vi "Begin.vi"(8 "error in":errorcluster) -> (0 "error out":errorcluster)   [LabVIEW 2019]
doc: "Called before other user functions, this VI can be used to open I/O refnums, load in file data, and do general program initialization. Notice that the <B>error out</B> terminal is simply used for data flow. Wiring it to other structures or subVIs ensures that this VI runs first."
uses:
  <vilib>/Rock Robotics/WPI/DriverStation/WPI_DriverStationRobotMode2.ctl
  <vilib>/Rock Robotics/WPI/Joystick/WPI_JoystickDeviceEnum.ctl
  <vilib>/Rock Robotics/SystemInterfaces/DIO/FPGA_DIOPWMChannel.ctl
  <vilib>/Rock Robotics/WPI/SafetyOutput/WPI_SafetyOutputConfigMenu.ctl
  <vilib>/Rock Robotics/WPI/Solenoid/WPI_SolenoidChannel.ctl
  <vilib>/Rock Robotics/WPI/Solenoid/WPI_SolenoidValue.ctl
  <vilib>/Rock Robotics/SystemInterfaces/i2clib/i2c_bus.ctl
  Robot Global Data.vi
  <vilib>/Rock Robotics/WPI/MotorControl/WPI_MotorControlOpen SPARK.vi
  <vilib>/Rock Robotics/WPI/Solenoid/WPI_SolenoidOpenDouble.vi
  <vilib>/Rock Robotics/WPI/Solenoid/WPI_SolenoidSetEnum.vi
  <vilib>/Rock Robotics/Network Tables/NT Write Number.vi
  <vilib>/Rock Robotics/WPI/RobotDrive/WPI_RobotDriveOpen2MotorWithExistingMotors.vi
  <vilib>/Rock Robotics/Network Tables/NT Write Numeric Array.vi
  <vilib>/Rock Robotics/Network Tables/NT Write Boolean Array.vi
panel:
  in  "Blue Calibration":cluster{"R":dbl, "G":dbl, "B":dbl}={"R"=0.143, "G"=0.427, "B"=0.429}
  in  "Green Calibration":cluster{"R":dbl, "G":dbl, "B":dbl}={"R"=0.197, "G"=0.561, "B"=0.24}
  in  "Red Calibration":cluster{"R":dbl, "G":dbl, "B":dbl}={"R"=0.561, "G"=0.323, "B"=0.114}
  in  "Yellow Calibration":cluster{"R":dbl, "G":dbl, "B":dbl}={"R"=0.361, "G"=0.524, "B"=0.113}
  in  "Calibration Time (sec)":u32=4
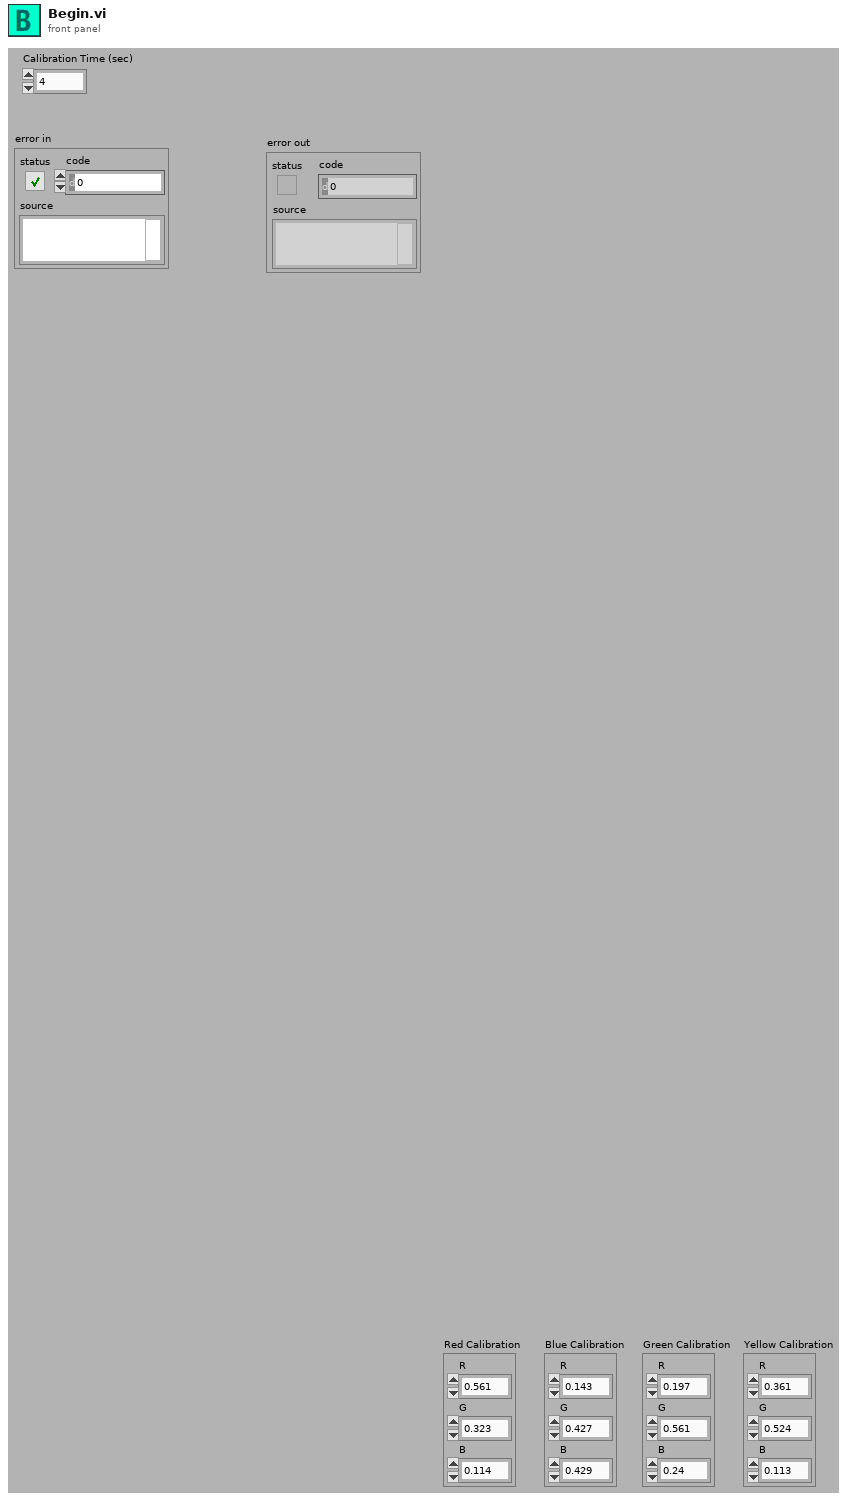
[diagram p1: front panel]
types:
  T1 = typedef "WPI_SolenoidChannel.ctl" = enum8{"Solenoid 0", "Solenoid 1", "Solenoid 2", "Solenoid 3", "Solenoid 4", "Solenoid 5", "Solenoid 6", "Solenoid 7", "Invalid"}
  T2 = typedef "WPI_SolenoidValue.ctl" = enum16{"Off", "On", "Forward", "Reverse"}
  T3 = typedef "WPI_SafetyOutputConfigMenu.ctl" = enum16{"Enable", "Disable"}
  T4 = typedef "i2c_bus.ctl" = enum16{"I2C On-Board", "I2C MXP", "Invalid"}
  T5 = typedef "FPGA_DIOPWMChannel.ctl" = enum8{"PWM 0", "PWM 1", "PWM 2", "PWM 3", "PWM 4", "PWM 5", "PWM 6", "PWM 7", "PWM 8", "PWM 9", "PWM MXP 0", "PWM MXP 1", "PWM MXP 2", "PWM MXP 3", "PWM MXP 4", "PWM MXP 5", "PWM MXP 6", "PWM MXP 7", "PWM MXP 8", "PWM MXP 9", "Invalid"}
  T6 = typedef "WPI_JoystickDeviceEnum.ctl" = enum16{"USB 0", "USB 1", "USB 2", "USB 3", "USB 4", "USB 5"}
  T7 = typedef "WPI_DriverStationRobotMode2.ctl" = enum16{"Autonomous Disabled", "Autonomous Enabled", "Teleop Disabled", "Teleop Enabled", "Disconnected", "Finish", "Test Disabled", "Test Enabled", "Emergency Stopped"}
  T8 = typedef "WPI_JoystickDevRef.ctl" = cluster{"Device":T6}
  T9 = typedef "WPI_MotorControlDeviceRef.ctl" = cluster{"DeviceStatus":errorcluster, "Type":T10, "PWM":cluster{"PWM Channel":T5, "DeadBand":T11}, "CAN":cluster{"Device Number":u8, "SetOutput VI Ref":variant, "GetOutput VI Ref":variant, "Enable VI Ref":variant, "Disable VI Ref":variant, "Data":variant}, "Invert":bool, "DIO PWM":cluster{"PWM \"Enable\" Channel":T5, "DIOChannel":T12, "PWM Rate":dbl}}
  T10 = typedef "WPI_MotorControlType.ctl" = enum16{"PWM", "CAN", "DIO PWM"}
  T11 = typedef "WPI_PWMDeadband.ctl" = cluster{"Name":string, "maxPositivePwm":i32, "minPositivePwm":i32, "centerPwm":i32, "maxNegativePwm":i32, "minNegativePwm":i32, "angularRange":u16}
  T12 = typedef "FPGA_DIOChannel.ctl" = enum8{"DIO 0", "DIO 1", "DIO 2", "DIO 3", "DIO 4", "DIO 5", "DIO 6", "DIO 7", "DIO 8", "DIO 9", "DIO MXP 0", "DIO MXP 1", "DIO MXP 2", "DIO MXP 3", "DIO MXP 4", "DIO MXP 5", "DIO MXP 6", "DIO MXP 7", "DIO MXP 8", "DIO MXP 9", "DIO MXP 10", "DIO MXP 11", "DIO MXP 12", "DIO MXP 13", "DIO MXP 14", "DIO MXP 15", "SPI Port CS1", "SPI Port CS2", "SPI Port CS3", "SPI Port MISO", "SPI Port MOSI", "Invalid"}
  T13 = typedef "WPI_RobotDriveDevRef.ctl" = cluster{"DevStatus":errorcluster, "Motors[]":T9[], "Square Inputs":bool, "Max Output":dbl}
  T14 = typedef "ADIS 16448 HW Configuration.ctl" = cluster{"SPI Clock Rate (Hz)":dbl, "IMU SPI Mode (3)":T15, "IMU Reset Pin":T12, "IMU SPI Bus":T16, "IMU Data Ready Pin":T12, "Stall Config":cluster{"Pow2BytesPerRead":u8, "StallTicks":u16, "CsToSclkTicks":u8}, "IMU Status LED Pin":T12}
  T15 = typedef "WPI_SPIMode.ctl" = enum16{"Mode 0 (Clk Idle Low,Sample on Leading)", "Mode 1 (Clk Idle Low,Sample on Trailing)", "Mode 2 (Clk Idle High,Sample on Leading)", "Mode 3 (Clk Idle High,Sample on Trailing)"}
  T16 = typedef "spi_bus.ctl" = enum16{"SPI On-Board, CS0", "SPI On-Board, CS1", "SPI On-Board, CS2", "SPI On-Board, CS3", "SPI MXP", "Invalid"}
  T17 = typedef "Color Sensor V3 DevRef.ctl" = cluster{"I2CDevRef":T18}
  T18 = typedef "WPI_I2CDevRef.ctl" = cluster{"DevStatus":errorcluster, "Device Address":u8, "Handle":i32, "I2C Bus":T4}
  T19 = typedef "WPI_SolenoidDevRef.ctl" = cluster{"DevStatus":errorcluster, "Pneumatics Control Module":u8, "Forward Solenoid Channel":T1, "Reverse Solenoid Channel":T1}
  T20 = typedef "ADIS16448 Device Reference.ctl" = cluster{"DevStatus":errorcluster, "Hardware Config":T21, "Calibration Complete":refnum<notifier>, "Status FIFO":refnum<k33>, "Last Value Reference":refnum<data-value>, "Sychronous Process VI":T22, "Cmd FIFO":refnum<k33>, "Source":T23, "Data FIFO":refnum<k33>, "IMU Status LED Pin":T12, "Calibration Time":u32}
  T21 = typedef "ADIS16448 Hardware Configuration.ctl" = cluster{"SPI Clock Rate (Hz)":dbl, "IMU SPI Mode (3)":T15, "IMU Reset Pin":T12, "IMU SPI Bus":T16, "IMU Data Ready Pin":T12, "Stall Config":cluster{"Pow2BytesPerRead":u8, "StallTicks":u16, "CsToSclkTicks":u8}, "IMU Status LED Pin":T12}
  T22 = typedef "ADIS16448 Process.ctl" = refnum<vi>
  T23 = typedef "FPGA_CounterEncoderSourceConvertionLVSourceType.ctl" = cluster{"DevStatus":errorcluster, "AnalogTriggerMode?":bool, "DigitalMode":cluster{"DIO Channel":T24}, "AnalogTriggerMode":cluster{"AnalogTriggerIndex":T25, "OutputType":T26}}
  T24 = typedef "FPGA_DIODigitalSourceChannel.ctl" = enum8{"DIO 0", "DIO 1", "DIO 2", "DIO 3", "DIO 4", "DIO 5", "DIO 6", "DIO 7", "DIO 8", "DIO 9", "DIO MXP 0", "DIO MXP 1", "DIO MXP 2", "DIO MXP 3", "DIO MXP 4", "DIO MXP 5", "DIO MXP 6", "DIO MXP 7", "DIO MXP 8", "DIO MXP 9", "DIO MXP 10", "DIO MXP 11", "DIO MXP 12", "DIO MXP 13", "DIO MXP 14", "DIO MXP 15", "SPI Port CS1", "SPI Port CS2", "SPI Port CS3", "SPI Port MISO", "SPI Port MOSI", "Disabled"}
  T25 = typedef "FPGA_AnalogTriggerIndex.ctl" = enum8{"Trig 0", "Trig 1", "Trig 2", "Trig 3", "Trig 4", "Trig 5", "Trig 6", "Trig 7", "Invalid"}
  T26 = typedef "FPGA_AnalogTriggerOutType.ctl" = enum16{"InWindow", "TriggerState", "Rising", "Falling"}
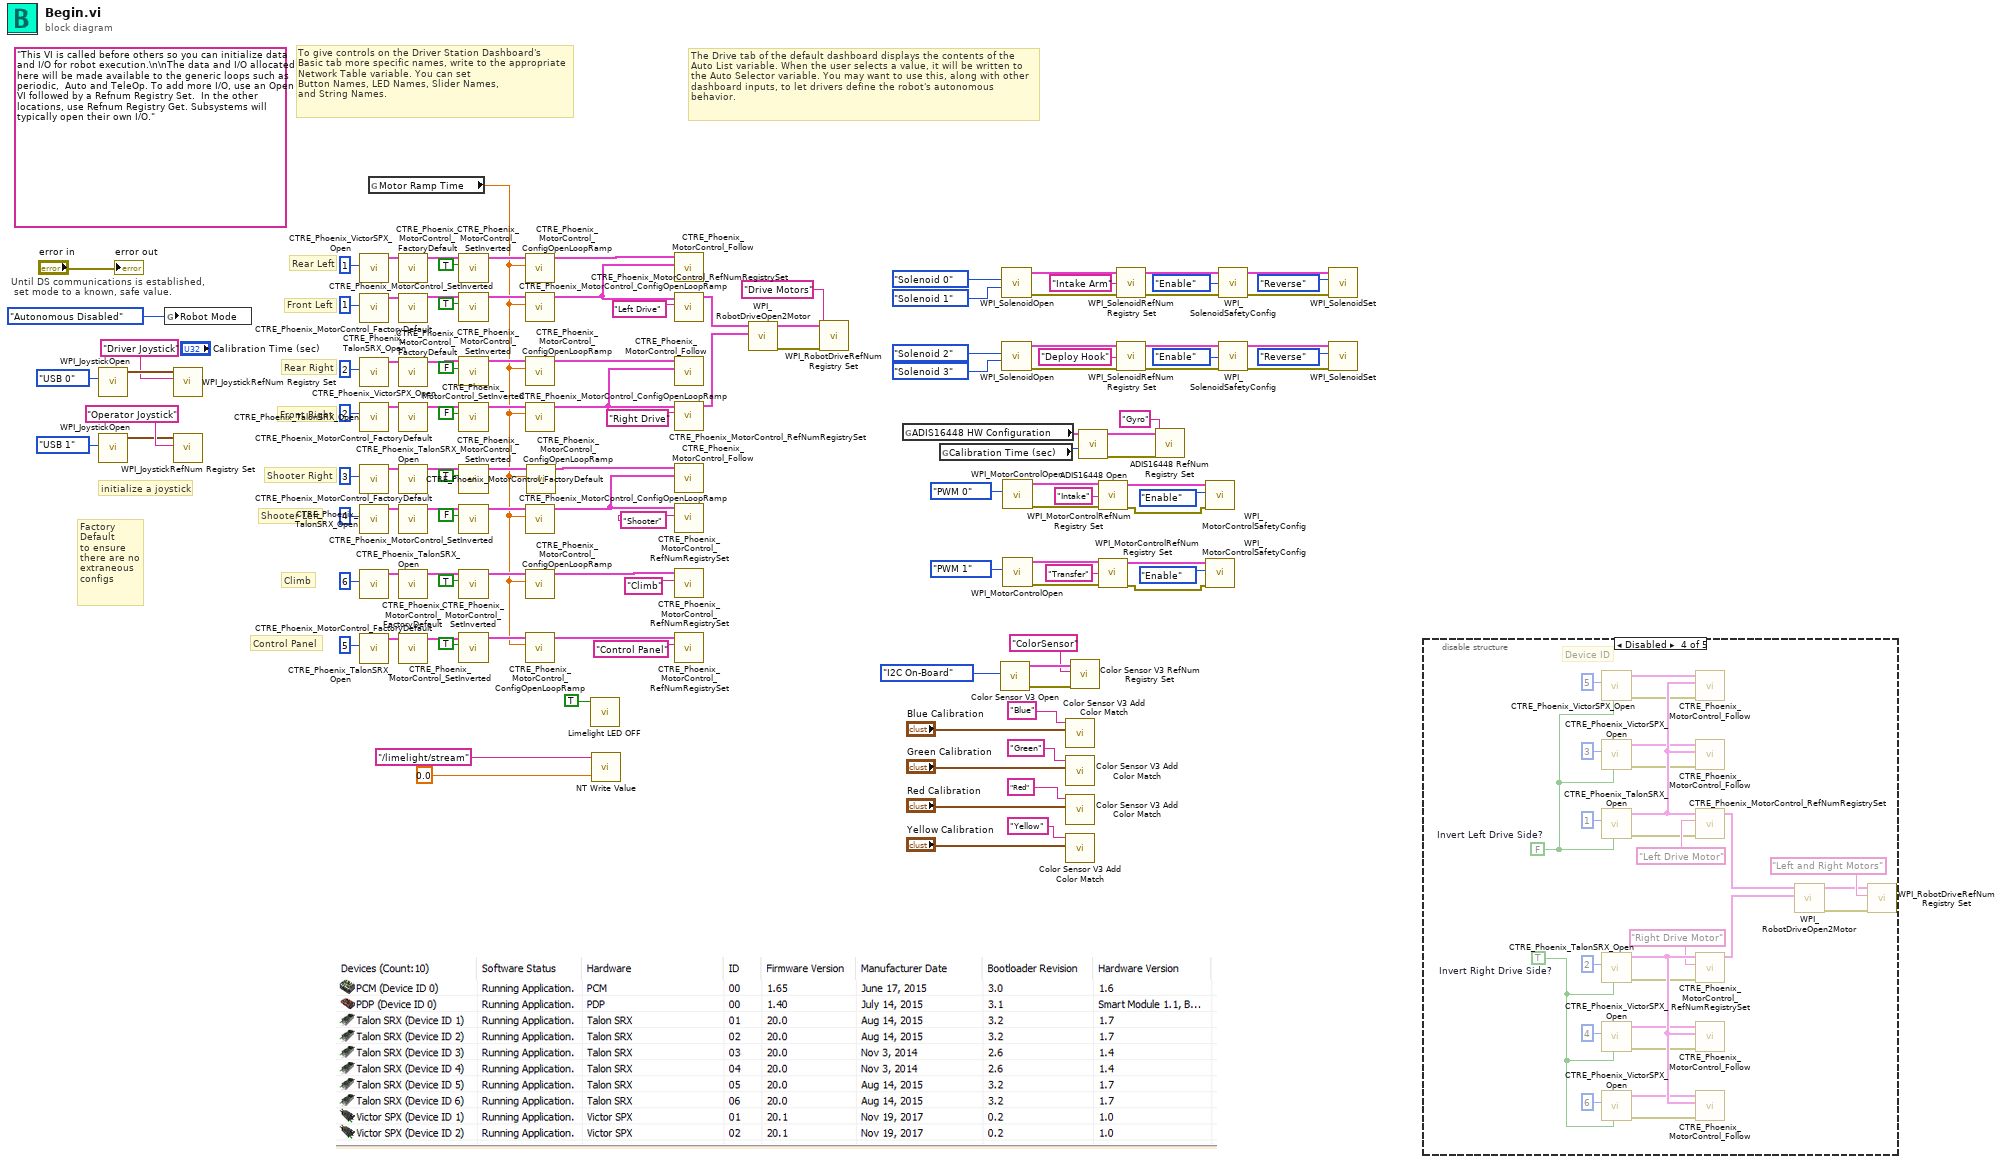
[diagram p0: block diagram]
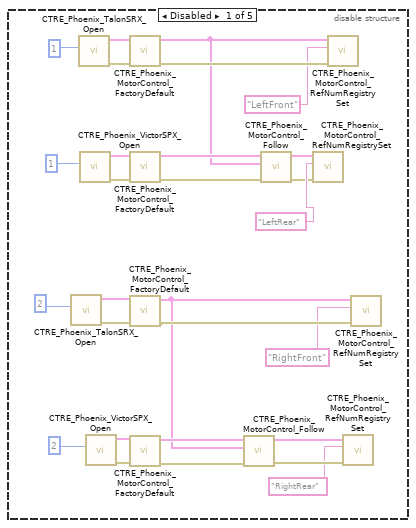
[diagram p2: hidden frame]
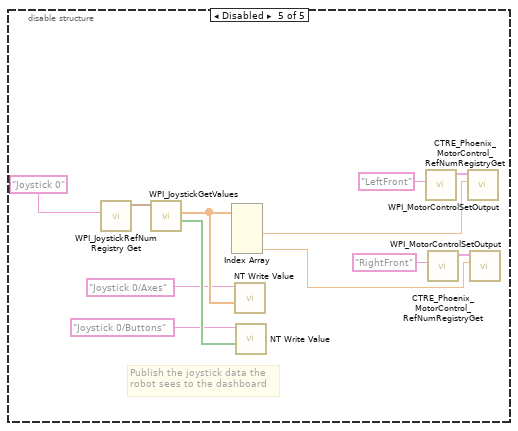
[diagram p5: hidden frame]
diagram:
  (unwired) "This VI is called before others so you can initialize data and I/O for robot execution.\n\nThe data and I/O allocated here will be made available to the generic loops such as periodic,  Auto and TeleOp. To add more I/O, use an Open VI followed by a Refnum Registry Set.  In the other locations, use Refnum Registry Get. Subsystems will typically open their own I/O."
  # "Climb"
  # "Control Panel"
  # "The Drive tab of the default dashboard displays the contents of the\nAuto List variable. When the user selects a value, it will be written to\nthe Auto Selector variable. You may want to use this, along with other\ndashboard inputs, to let drivers define the robot's autonomous\nbehavior."
  # "To give controls on the Driver Station Dashboard's\nBasic tab more specific names, write to the appropriate\nNetwork Table variable. You can set\nButton Names, LED Names, Slider Names,\nand String Names."
  # "Shooter Left"
  # "Shooter Right"
  # "Factory \nDefault \nto ensure \nthere are no \nextraneous \nconfigs"
  # "Front Right"
  # "Front Left"
  # "Rear Right"
  # "Rear Left"
  # "initialize a joystick"
  # "Until DS communications is established,\n set mode to a known, safe value."
  n1 = call <vilib>:"WPI_JoystickOpen.vi"("JoystickDevice"=WPI_JoystickDeviceEnum."USB 0") -> ("JoystickDevRef"=w106:T8)  [unwired: 10 in]
  n2 = call <vilib>:"WPI_JoystickOpen.vi"("JoystickDevice"=WPI_JoystickDeviceEnum."USB 1") -> ("JoystickDevRef"=w121:T8)  [unwired: 10 in]
  n3 = global write "Robot Global Data.vi" "Robot Mode"(WPI_DriverStationRobotMode2."Autonomous Disabled" ("Robot Mode")) -> ()
  n4 = call <vilib>:"WPI_JoystickRefNum Registry Set.vi"("refnum name"="Driver Joystick", "JoystickDevRef"=w106) -> ()  [unwired: 8 in, 2 out]
  n5 = call <vilib>:"WPI_JoystickRefNum Registry Set.vi"("refnum name"="Operator Joystick", "JoystickDevRef"=w121) -> ()  [unwired: 8 in, 2 out]
  n6 = call <vilib>:"CTRE_Phoenix_VictorSPX_Open.vi"("Device Number"=u8 1) -> ("CAN Talon SRX Ref"=w104:T9)  [unwired: 9 in, 1 out]
  n7 = call <vilib>:"CTRE_Phoenix_TalonSRX_Open.vi"("Device Number"=u8 1) -> ("CAN Talon SRX Ref"=w103:T9)  [unwired: 9 in, 1 out]
  n8 = call <vilib>:"CTRE_Phoenix_VictorSPX_Open.vi"("Device Number"=u8 2) -> ("CAN Talon SRX Ref"=w102:T9)  [unwired: 9 in, 1 out]
  n9 = call <vilib>:"CTRE_Phoenix_TalonSRX_Open.vi"("Device Number"=u8 2) -> ("CAN Talon SRX Ref"=w101:T9)  [unwired: 9 in, 1 out]
  n10 = call <vilib>:"CTRE_Phoenix_TalonSRX_Open.vi"("Device Number"=u8 3) -> ("CAN Talon SRX Ref"=w75:T9)  [unwired: 9 in, 1 out]
  n11 = call <vilib>:"CTRE_Phoenix_TalonSRX_Open.vi"("Device Number"=u8 4) -> ("CAN Talon SRX Ref"=w74:T9)  [unwired: 9 in, 1 out]
  n12 = call <vilib>:"CTRE_Phoenix_TalonSRX_Open.vi"("Device Number"=u8 6) -> ("CAN Talon SRX Ref"=w26:T9)  [unwired: 9 in, 1 out]
  n13 = call <vilib>:"CTRE_Phoenix_TalonSRX_Open.vi"("Device Number"=u8 5) -> ("CAN Talon SRX Ref"=w56:T9)  [unwired: 9 in, 1 out]
  n14 = global read "Robot Global Data.vi" "Motor Ramp Time"() -> (w1:dbl)
  n15 = call <vilib>:"CTRE_Phoenix_MotorControl_FactoryDefault.vi"("PhoenixMotorControlDevRef"=w104) -> ("PhoenixMotorControlDevRef"=w99:T9)  [unwired: 9 in, 1 out]
  n16 = call <vilib>:"CTRE_Phoenix_MotorControl_FactoryDefault.vi"("PhoenixMotorControlDevRef"=w103) -> ("PhoenixMotorControlDevRef"=w97:T9)  [unwired: 9 in, 1 out]
  n17 = call <vilib>:"CTRE_Phoenix_MotorControl_FactoryDefault.vi"("PhoenixMotorControlDevRef"=w102) -> ("PhoenixMotorControlDevRef"=w95:T9)  [unwired: 9 in, 1 out]
  n18 = call <vilib>:"CTRE_Phoenix_MotorControl_FactoryDefault.vi"("PhoenixMotorControlDevRef"=w101) -> ("PhoenixMotorControlDevRef"=w93:T9)  [unwired: 9 in, 1 out]
  n19 = call <vilib>:"CTRE_Phoenix_MotorControl_FactoryDefault.vi"("PhoenixMotorControlDevRef"=w75) -> ("PhoenixMotorControlDevRef"=w72:T9)  [unwired: 9 in, 1 out]
  n20 = call <vilib>:"CTRE_Phoenix_MotorControl_FactoryDefault.vi"("PhoenixMotorControlDevRef"=w74) -> ("PhoenixMotorControlDevRef"=w70:T9)  [unwired: 9 in, 1 out]
  n21 = call <vilib>:"CTRE_Phoenix_MotorControl_FactoryDefault.vi"("PhoenixMotorControlDevRef"=w26) -> ("PhoenixMotorControlDevRef"=w24:T9)  [unwired: 9 in, 1 out]
  n22 = call <vilib>:"CTRE_Phoenix_MotorControl_FactoryDefault.vi"("PhoenixMotorControlDevRef"=w56) -> ("PhoenixMotorControlDevRef"=w54:T9)  [unwired: 9 in, 1 out]
  n23 = call <vilib>:"CTRE_Phoenix_MotorControl_SetInverted.vi"("Invert?"=TRUE, "PhoenixMotorControlDevRef"=w99) -> ("PhoenixMotorControlDevRef"=w17:T9)  [unwired: 8 in, 1 out]
  n24 = call <vilib>:"CTRE_Phoenix_MotorControl_SetInverted.vi"("Invert?"=TRUE, "PhoenixMotorControlDevRef"=w97) -> ("PhoenixMotorControlDevRef"=w15:T9)  [unwired: 8 in, 1 out]
  n25 = call <vilib>:"CTRE_Phoenix_MotorControl_SetInverted.vi"("Invert?"=FALSE, "PhoenixMotorControlDevRef"=w95) -> ("PhoenixMotorControlDevRef"=w9:T9)  [unwired: 8 in, 1 out]
  n26 = call <vilib>:"CTRE_Phoenix_MotorControl_SetInverted.vi"("Invert?"=FALSE, "PhoenixMotorControlDevRef"=w93) -> ("PhoenixMotorControlDevRef"=w10:T9)  [unwired: 8 in, 1 out]
  n27 = call <vilib>:"CTRE_Phoenix_MotorControl_SetInverted.vi"("Invert?"=TRUE, "PhoenixMotorControlDevRef"=w72) -> ("PhoenixMotorControlDevRef"=w3:T9)  [unwired: 8 in, 1 out]
  n28 = call <vilib>:"CTRE_Phoenix_MotorControl_SetInverted.vi"("Invert?"=FALSE, "PhoenixMotorControlDevRef"=w70) -> ("PhoenixMotorControlDevRef"=w11:T9)  [unwired: 8 in, 1 out]
  n29 = call <vilib>:"CTRE_Phoenix_MotorControl_SetInverted.vi"("Invert?"=TRUE, "PhoenixMotorControlDevRef"=w24) -> ("PhoenixMotorControlDevRef"=w12:T9)  [unwired: 8 in, 1 out]
  n30 = call <vilib>:"CTRE_Phoenix_MotorControl_SetInverted.vi"("Invert?"=TRUE, "PhoenixMotorControlDevRef"=w54) -> ("PhoenixMotorControlDevRef"=w13:T9)  [unwired: 8 in, 1 out]
  n31 = call <vilib>:"CTRE_Phoenix_MotorControl_ConfigOpenLoopRamp.vi"("secondsFromNeutralToFull"=w1, "PhoenixMotorControlDevRef"=w17) -> ("PhoenixMotorControlDevRef"=w16:T9)  [unwired: 8 in, 1 out]
  n32 = call <vilib>:"CTRE_Phoenix_MotorControl_ConfigOpenLoopRamp.vi"("secondsFromNeutralToFull"=w1, "PhoenixMotorControlDevRef"=w15) -> ("PhoenixMotorControlDevRef"=w14:T9)  [unwired: 8 in, 1 out]
  n33 = call <vilib>:"CTRE_Phoenix_MotorControl_ConfigOpenLoopRamp.vi"("secondsFromNeutralToFull"=w1, "PhoenixMotorControlDevRef"=w9) -> ("PhoenixMotorControlDevRef"=w8:T9)  [unwired: 8 in, 1 out]
  n34 = call <vilib>:"CTRE_Phoenix_MotorControl_ConfigOpenLoopRamp.vi"("secondsFromNeutralToFull"=w1, "PhoenixMotorControlDevRef"=w10) -> ("PhoenixMotorControlDevRef"=w7:T9)  [unwired: 8 in, 1 out]
  n35 = call <vilib>:"CTRE_Phoenix_MotorControl_ConfigOpenLoopRamp.vi"("secondsFromNeutralToFull"=w1, "PhoenixMotorControlDevRef"=w11) -> ("PhoenixMotorControlDevRef"=w6:T9)  [unwired: 8 in, 1 out]
  n36 = call <vilib>:"CTRE_Phoenix_MotorControl_ConfigOpenLoopRamp.vi"("secondsFromNeutralToFull"=w1, "PhoenixMotorControlDevRef"=w12) -> ("PhoenixMotorControlDevRef"=w5:T9)  [unwired: 8 in, 1 out]
  n37 = call <vilib>:"CTRE_Phoenix_MotorControl_ConfigOpenLoopRamp.vi"("secondsFromNeutralToFull"=w1, "PhoenixMotorControlDevRef"=w13) -> ("PhoenixMotorControlDevRef"=w4:T9)  [unwired: 8 in, 1 out]
  n38 = call <vilib>:"CTRE_Phoenix_MotorControl_ConfigOpenLoopRamp.vi"("secondsFromNeutralToFull"=w1, "PhoenixMotorControlDevRef"=w3) -> ("PhoenixMotorControlDevRef"=w2:T9)  [unwired: 8 in, 1 out]
  n39 = call "Limelight LED OFF.vi"("D Select  8"=TRUE) -> ()  [unwired: 10 in, 1 out]
  n40 = call-poly <vilib>:"NT Write Value.vi"("Numeric"=0.0, "Name"="/limelight/stream") -> ()  [unwired: 9 in, 1 out]
  n41 = call <vilib>:"CTRE_Phoenix_MotorControl_Follow.vi"("Master Controller to Follow"=w14, "PhoenixMotorControlDevRef"=w16) -> ()  [unwired: 8 in, 2 out]
  n42 = call <vilib>:"CTRE_Phoenix_MotorControl_RefNumRegistrySet.vi"("refnum name"="Left Drive", "PhoenixMotorControlDevRef"=w14) -> ("PhoenixMotorControlDevRef"=w114:T9)  [unwired: 8 in, 1 out]
  n43 = call <vilib>:"CTRE_Phoenix_MotorControl_Follow.vi"("Master Controller to Follow"=w7, "PhoenixMotorControlDevRef"=w8) -> ()  [unwired: 8 in, 2 out]
  n44 = call <vilib>:"CTRE_Phoenix_MotorControl_RefNumRegistrySet.vi"("refnum name"="Right Drive", "PhoenixMotorControlDevRef"=w7) -> ("PhoenixMotorControlDevRef"=w113:T9)  [unwired: 8 in, 1 out]
  n45 = call <vilib>:"CTRE_Phoenix_MotorControl_Follow.vi"("Master Controller to Follow"=w6, "PhoenixMotorControlDevRef"=w2) -> ()  [unwired: 8 in, 2 out]
  n46 = call <vilib>:"CTRE_Phoenix_MotorControl_RefNumRegistrySet.vi"("refnum name"="Shooter", "PhoenixMotorControlDevRef"=w6) -> ()  [unwired: 8 in, 2 out]
  n47 = call <vilib>:"CTRE_Phoenix_MotorControl_RefNumRegistrySet.vi"("refnum name"="Climb", "PhoenixMotorControlDevRef"=w5) -> ()  [unwired: 8 in, 2 out]
  n48 = call <vilib>:"CTRE_Phoenix_MotorControl_RefNumRegistrySet.vi"("refnum name"="Control Panel", "PhoenixMotorControlDevRef"=w4) -> ()  [unwired: 8 in, 2 out]
  n49 = call-poly <vilib>:"WPI_RobotDriveOpen2Motor.vi"("Right Motor Dev Ref"=w113, "Left Motor Dev Ref"=w114) -> ("error out"=w109:errorcluster, "RobotDriveDevRef"=w110:T13)  [unwired: 8 in]
  n50 = call <vilib>:"WPI_RobotDriveRefNum Registry Set.vi"("error in (no error)"=w109, "refnum name"="Drive Motors", "RobotDriveDevRef"=w110) -> ()  [unwired: 7 in, 2 out]
  n51 = global read "Robot Global Data.vi" "ADIS16448 HW Configuration"() -> (w22:T14)
  n52 = global read "Robot Global Data.vi" "Calibration Time (sec)"() -> (w21:u32)
  n53 = call <vilib>:"Color Sensor V3 Open.vi"("I2C Bus"=i2c_bus."I2C On-Board") -> ("error out"=w51:errorcluster, "ColorSensorDevRef"=w52:T17)  [unwired: 9 in]
  n54 = call-poly <vilib>:"WPI_SolenoidOpen.vi"("Reverse Solenoid Channel"=WPI_SolenoidChannel."Solenoid 1" ("Solenoid Channel"), "Forward Solenoid Channel"=WPI_SolenoidChannel."Solenoid 0" ("Solenoid Channel")) -> ("error out"=w66:errorcluster, "SolenoidDevRef"=w69:T19)  [unwired: 8 in]
  n55 = call-poly <vilib>:"WPI_SolenoidOpen.vi"("Reverse Solenoid Channel"=WPI_SolenoidChannel."Solenoid 3" ("Solenoid Channel"), "Forward Solenoid Channel"=WPI_SolenoidChannel."Solenoid 2" ("Solenoid Channel")) -> ("error out"=w33:errorcluster, "SolenoidDevRef"=w30:T19)  [unwired: 8 in]
  n56 = call-poly <vilib>:"WPI_MotorControlOpen.vi"("PWM Channel"=FPGA_DIOPWMChannel."PWM 0") -> ("error out"=w87:errorcluster, "MotorControlDeviceRef"=w91:T9)  [unwired: 9 in]
  n57 = call-poly <vilib>:"WPI_MotorControlOpen.vi"("PWM Channel"=FPGA_DIOPWMChannel."PWM 1") -> ("error out"=w84:errorcluster, "MotorControlDeviceRef"=w80:T9)  [unwired: 9 in]
  n58 = call <vilib>:"Color Sensor V3 Add Color Match.vi"("Color"="Blue Calibration", "Name"="Blue") -> ()  [unwired: 10 in]
  n59 = call <vilib>:"Color Sensor V3 Add Color Match.vi"("Color"="Green Calibration", "Name"="Green") -> ()  [unwired: 10 in]
  n60 = call <vilib>:"Color Sensor V3 Add Color Match.vi"("Color"="Red Calibration", "Name"="Red") -> ()  [unwired: 10 in]
  n61 = call <vilib>:"Color Sensor V3 Add Color Match.vi"("Color"="Yellow Calibration", "Name"="Yellow") -> ()  [unwired: 10 in]
  n62 = call <vilib>:"Color Sensor V3 RefNum Registry Set.vi"("error in (no error)"=w51, "refnum name"="ColorSensor", "ColorSensorDevRef"=w52) -> ()  [unwired: 7 in, 2 out]
  n63 = call <vilib>:"ADIS16448 Open.vi"("Initial Calibration Time (sec)"=w21, "Hardware Config"=w22) -> ("error out"=w19:errorcluster, "ADIS16448DevRef"=w20:T20)  [unwired: 8 in]
  n64 = call <vilib>:"WPI_MotorControlRefNum Registry Set.vi"("error in (no error)"=w87, "refnum name"="Intake", "MotorControlDevRef"=w91) -> ("error out"=w86:errorcluster, "MotorControlDevRef"=w90:T9)  [unwired: 7 in]
  n65 = call <vilib>:"WPI_MotorControlRefNum Registry Set.vi"("error in (no error)"=w84, "refnum name"="Transfer", "MotorControlDevRef"=w80) -> ("error out"=w85:errorcluster, "MotorControlDevRef"=w81:T9)  [unwired: 7 in]
  n66 = call <vilib>:"WPI_SolenoidRefNum Registry Set.vi"("error in (no error)"=w66, "refnum name"="Intake Arm", "SolenoidDevRef"=w69) -> ("error out"=w65:errorcluster, "SolenoidDevRef"=w68:T19)  [unwired: 7 in]
  n67 = call <vilib>:"WPI_SolenoidRefNum Registry Set.vi"("error in (no error)"=w33, "refnum name"="Deploy Hook", "SolenoidDevRef"=w30) -> ("error out"=w34:errorcluster, "SolenoidDevRef"=w31:T19)  [unwired: 7 in]
  n68 = call <vilib>:"ADIS16448 RefNum Registry Set.vi"("error in (no error)"=w19, "refnum name"="Gyro", "ADIS16448DevRef"=w20) -> ()  [unwired: 7 in, 2 out]
  n69 = call <vilib>:"WPI_MotorControlSafetyConfig.vi"("error in (no error)"=w86, "mode"=WPI_SafetyOutputConfigMenu."Enable", "MotorControlDevRef"=w90) -> ()  [unwired: 7 in, 2 out]
  n70 = call <vilib>:"WPI_MotorControlSafetyConfig.vi"("error in (no error)"=w85, "mode"=WPI_SafetyOutputConfigMenu."Enable", "MotorControlDevRef"=w81) -> ()  [unwired: 7 in, 2 out]
  n71 = call <vilib>:"WPI_SolenoidSafetyConfig.vi"("error in (no error)"=w65, "mode"=WPI_SafetyOutputConfigMenu."Enable", "SolenoidDevRef"=w68) -> ("error out"=w64:errorcluster, "SolenoidDevRef"=w67:T19)  [unwired: 7 in]
  n72 = call <vilib>:"WPI_SolenoidSafetyConfig.vi"("error in (no error)"=w34, "mode"=WPI_SafetyOutputConfigMenu."Enable", "SolenoidDevRef"=w31) -> ("error out"=w35:errorcluster, "SolenoidDevRef"=w32:T19)  [unwired: 7 in]
  n73 = call-poly <vilib>:"WPI_SolenoidSet.vi"("error in (no error)"=w64, "Value"=WPI_SolenoidValue."Reverse", "SolenoidDevRef"=w67) -> ()  [unwired: 7 in, 2 out]
  n74 = call-poly <vilib>:"WPI_SolenoidSet.vi"("error in (no error)"=w35, "Value"=WPI_SolenoidValue."Reverse", "SolenoidDevRef"=w32) -> ()  [unwired: 7 in, 2 out]
  n75 = disable-structure shown="Disabled" {
    frame Disabled {
      n76 = call <vilib>:"CTRE_Phoenix_TalonSRX_Open.vi"("Device Number"=u8 2) -> ("error out"=w148:errorcluster, "CAN Talon SRX Ref"=w138:T9)  [unwired: 9 in]
      n77 = call <vilib>:"CTRE_Phoenix_TalonSRX_Open.vi"("Device Number"=u8 1) -> ("error out"=w146:errorcluster, "CAN Talon SRX Ref"=w136:T9)  [unwired: 9 in]
      n78 = call <vilib>:"CTRE_Phoenix_VictorSPX_Open.vi"("Device Number"=u8 1) -> ("error out"=w144:errorcluster, "CAN Talon SRX Ref"=w142:T9)  [unwired: 9 in]
      n79 = call <vilib>:"CTRE_Phoenix_VictorSPX_Open.vi"("Device Number"=u8 2) -> ("error out"=w150:errorcluster, "CAN Talon SRX Ref"=w140:T9)  [unwired: 9 in]
      n80 = call <vilib>:"CTRE_Phoenix_MotorControl_FactoryDefault.vi"("error in"=w146, "PhoenixMotorControlDevRef"=w136) -> ("error out"=w147:errorcluster, "PhoenixMotorControlDevRef"=w137:T9)  [unwired: 8 in]
      n81 = call <vilib>:"CTRE_Phoenix_MotorControl_FactoryDefault.vi"("error in"=w144, "PhoenixMotorControlDevRef"=w142) -> ("error out"=w145:errorcluster, "PhoenixMotorControlDevRef"=w143:T9)  [unwired: 8 in]
      n82 = call <vilib>:"CTRE_Phoenix_MotorControl_FactoryDefault.vi"("error in"=w148, "PhoenixMotorControlDevRef"=w138) -> ("error out"=w149:errorcluster, "PhoenixMotorControlDevRef"=w139:T9)  [unwired: 8 in]
      n83 = call <vilib>:"CTRE_Phoenix_MotorControl_FactoryDefault.vi"("error in"=w150, "PhoenixMotorControlDevRef"=w140) -> ("error out"=w151:errorcluster, "PhoenixMotorControlDevRef"=w141:T9)  [unwired: 8 in]
      n84 = call <vilib>:"CTRE_Phoenix_MotorControl_Follow.vi"("error in (no error)"=w151, "Master Controller to Follow"=w139, "PhoenixMotorControlDevRef"=w141) -> ("error out"=w134:errorcluster, "PhoenixMotorControlDevRef"=w135:T9)  [unwired: 7 in]
      n85 = call <vilib>:"CTRE_Phoenix_MotorControl_Follow.vi"("error in (no error)"=w145, "Master Controller to Follow"=w137, "PhoenixMotorControlDevRef"=w143) -> ("error out"=w126:errorcluster, "PhoenixMotorControlDevRef"=w127:T9)  [unwired: 7 in]
      n86 = call <vilib>:"CTRE_Phoenix_MotorControl_RefNumRegistrySet.vi"("error in (no error)"=w126, "refnum name"="LeftRear", "PhoenixMotorControlDevRef"=w127) -> ()  [unwired: 7 in, 2 out]
      n87 = call <vilib>:"CTRE_Phoenix_MotorControl_RefNumRegistrySet.vi"("error in (no error)"=w147, "refnum name"="LeftFront", "PhoenixMotorControlDevRef"=w137) -> ()  [unwired: 7 in, 2 out]
      n88 = call <vilib>:"CTRE_Phoenix_MotorControl_RefNumRegistrySet.vi"("error in (no error)"=w134, "refnum name"="RightRear", "PhoenixMotorControlDevRef"=w135) -> ()  [unwired: 7 in, 2 out]
      n89 = call <vilib>:"CTRE_Phoenix_MotorControl_RefNumRegistrySet.vi"("error in (no error)"=w149, "refnum name"="RightFront", "PhoenixMotorControlDevRef"=w139) -> ()  [unwired: 7 in, 2 out]
    }
    frame Enabled {
    }
    frame Disabled {
    }
    frame Disabled {
      w178 = FALSE  # Invert Left Drive Side?
      w177 = TRUE  # Invert Right Drive Side?
      # "Device ID"
      n90 = call <vilib>:"CTRE_Phoenix_VictorSPX_Open.vi"("Invert"=w178, "Device Number"=u8 5) -> ("error out"=w168:errorcluster, "CAN Talon SRX Ref"=w169:T9)  [unwired: 8 in]
      n91 = call <vilib>:"CTRE_Phoenix_VictorSPX_Open.vi"("Invert"=w178, "Device Number"=u8 3) -> ("error out"=w167:errorcluster, "CAN Talon SRX Ref"=w170:T9)  [unwired: 8 in]
      n92 = call <vilib>:"CTRE_Phoenix_TalonSRX_Open.vi"("Invert"=w178, "Device Number"=u8 1) -> ("error out"=w158:errorcluster, "CAN Talon SRX Ref"=w171:T9)  [unwired: 8 in]
      n93 = call <vilib>:"CTRE_Phoenix_TalonSRX_Open.vi"("Invert"=w177, "Device Number"=u8 2) -> ("error out"=w159:errorcluster, "CAN Talon SRX Ref"=w166:T9)  [unwired: 8 in]
      n94 = call <vilib>:"CTRE_Phoenix_VictorSPX_Open.vi"("Invert"=w177, "Device Number"=u8 4) -> ("error out"=w162:errorcluster, "CAN Talon SRX Ref"=w163:T9)  [unwired: 8 in]
      n95 = call <vilib>:"CTRE_Phoenix_VictorSPX_Open.vi"("Invert"=w177, "Device Number"=u8 6) -> ("error out"=w165:errorcluster, "CAN Talon SRX Ref"=w164:T9)  [unwired: 8 in]
      n96 = call <vilib>:"CTRE_Phoenix_MotorControl_Follow.vi"("error in (no error)"=w168, "Master Controller to Follow"=w171, "PhoenixMotorControlDevRef"=w169) -> ()  [unwired: 7 in, 2 out]
      n97 = call <vilib>:"CTRE_Phoenix_MotorControl_Follow.vi"("error in (no error)"=w167, "Master Controller to Follow"=w171, "PhoenixMotorControlDevRef"=w170) -> ()  [unwired: 7 in, 2 out]
      n98 = call <vilib>:"CTRE_Phoenix_MotorControl_RefNumRegistrySet.vi"("error in (no error)"=w158, "refnum name"="Left Drive Motor", "PhoenixMotorControlDevRef"=w171) -> ("PhoenixMotorControlDevRef"=w172:T9)  [unwired: 7 in, 1 out]
      n99 = call <vilib>:"CTRE_Phoenix_MotorControl_RefNumRegistrySet.vi"("error in (no error)"=w159, "refnum name"="Right Drive Motor", "PhoenixMotorControlDevRef"=w166) -> ("PhoenixMotorControlDevRef"=w173:T9)  [unwired: 7 in, 1 out]
      n100 = call <vilib>:"CTRE_Phoenix_MotorControl_Follow.vi"("error in (no error)"=w162, "Master Controller to Follow"=w166, "PhoenixMotorControlDevRef"=w163) -> ()  [unwired: 7 in, 2 out]
      n101 = call <vilib>:"CTRE_Phoenix_MotorControl_Follow.vi"("error in (no error)"=w165, "Master Controller to Follow"=w166, "PhoenixMotorControlDevRef"=w164) -> ()  [unwired: 7 in, 2 out]
      n102 = call-poly <vilib>:"WPI_RobotDriveOpen2Motor.vi"("Right Motor Dev Ref"=w173, "Left Motor Dev Ref"=w172) -> ("error out"=w174:errorcluster, "RobotDriveDevRef"=w175:T13)  [unwired: 8 in]
      n103 = call <vilib>:"WPI_RobotDriveRefNum Registry Set.vi"("error in (no error)"=w174, "refnum name"="Left and Right Motors", "RobotDriveDevRef"=w175) -> ()  [unwired: 7 in, 2 out]
    }
    frame Disabled {
      # "Publish the joystick data the\nrobot sees to the dashboard"
      n104 = call <vilib>:"WPI_JoystickRefNum Registry Get.vi"("refnum name"="Joystick 0") -> ("JoystickDevRef"=w180:T8)  [unwired: 1 in, 9 out]
      n105 = call <vilib>:"WPI_JoystickGetValues.vi"("JoystickDevRef"=w180) -> ("Buttons"=w184:bool[], "Axes"=w183:dbl[])  [unwired: 6 in, 3 out]
      n106 = Index Array(array=w183) -> (element #2=w187:dbl, element #4=w190:dbl)  [unwired: 4 in, 2 out]
      n107 = call-poly <vilib>:"NT Write Value.vi"("Numeric Array"=w183, "Name"="Joystick 0/Axes") -> ()  [unwired: 9 in, 1 out]
      n108 = call-poly <vilib>:"NT Write Value.vi"("Boolean Array"=w184, "Name"="Joystick 0/Buttons") -> ()  [unwired: 9 in, 1 out]
      n109 = call <vilib>:"CTRE_Phoenix_MotorControl_RefNumRegistryGet.vi"("refnum name"="LeftFront") -> ("PhoenixMotorControlDevRef"=w186:T9)  [unwired: 9 in, 1 out]
      n110 = call <vilib>:"CTRE_Phoenix_MotorControl_RefNumRegistryGet.vi"("refnum name"="RightFront") -> ("PhoenixMotorControlDevRef"=w189:T9)  [unwired: 9 in, 1 out]
      n111 = call <vilib>:"WPI_MotorControlSetOutput.vi"("Output"=w187, "MotorControlDevRef"=w186) -> ()  [unwired: 7 in, 3 out]
      n112 = call <vilib>:"WPI_MotorControlSetOutput.vi"("Output"=w190, "MotorControlDevRef"=w189) -> ()  [unwired: 7 in, 3 out]
    }
  }
  "error out" <- "error in"
